vi "Endpoint Connected.vi"(8 "error in (no error)":errorcluster, 10 "Endpoint":refnum<class "Message Enqueuer.lvclass">, 11 "MSS Host Actor in":refnum<class "MSS Host Actor.lvclass">) -> (0 "error out":errorcluster, 3 "MSS Host Actor out":refnum<class "MSS Host Actor.lvclass">)   [LabVIEW 2023, in "MSS Host Actor.lvlib" / "MSS Host Actor.lvclass"]
doc: "Override this method to specify how the receiving actor responds to a Connected message from a nested endpoint actor."
uses:
  <vilib>/ActorFramework/Message Enqueuer/Message Enqueuer.lvclass
  MSS Host Actor.lvclass
  MSS Host Actor.lvclass/MSS Host Actor.ctl
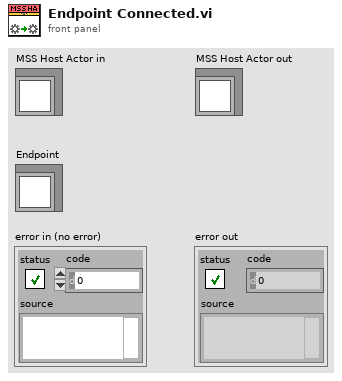
[diagram p1: front panel]
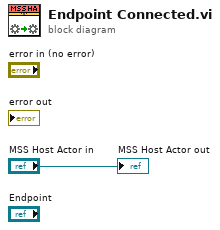
[diagram p0: block diagram]
diagram:
  "MSS Host Actor out" <- "MSS Host Actor in"
